vi "Set Theme.vi"(10 "Dark?":bool, 11 "VI in":refnum<vi>) -> ()   [LabVIEW 2019, in "Panther Dashboard.lvlib"]
uses:
  Panther Dashboard.lvlib
  <vilib>/Utility/miscctls.llb/LVTextColorsTypeDef.ctl
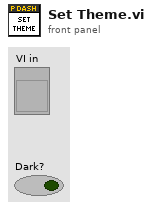
[diagram p1: front panel]
types:
  T1 = typedef "LVTextColorsTypeDef.ctl" = cluster{"Text Color":u32, "Background Color":u32}
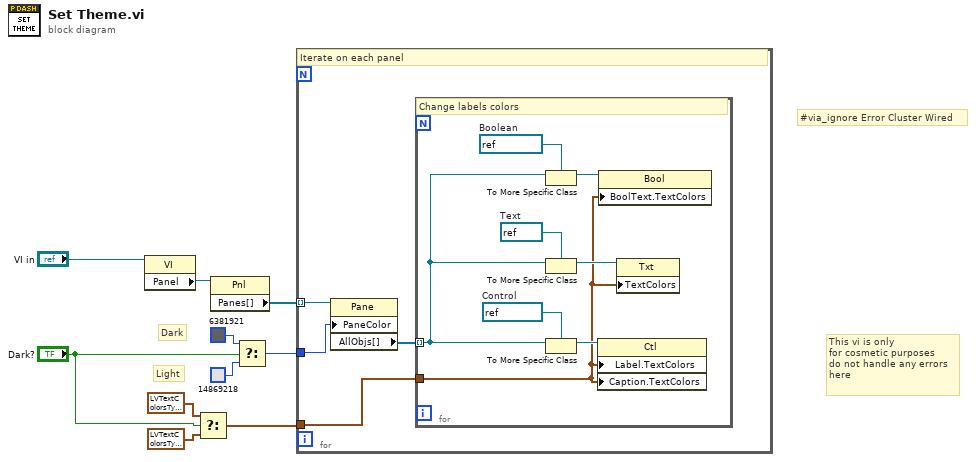
[diagram p0: block diagram]
diagram:
  # "#via_ignore Error Cluster Wired"
  # "This vi is only \nfor cosmetic purposes\ndo not handle any errors\nhere"
  # "Light"
  # "Dark"
  n1 = property class="VI"(reference="VI in") -> ("Panel"=w5:refnum<vi>)  [unwired: 1 in, 2 out]
  n2 = Select(t=T1 {"Text Color"=16448250, "Background Color"=16777216} ("Label.Text Colors"), s="Dark?", f=T1 {"Text Color"=0, "Background Color"=16777216} ("Label.Text Colors")) -> (s? t:f=w2:T1)
  n3 = property class="Pnl"(reference=w5) -> ("Panes[]"=w4:refnum<vi>[])  [unwired: 1 in, 2 out]
  n4 = Select(t=u32 6381921, s="Dark?", f=u32 14869218) -> (s? t:f=w3:u32)
  n5 = for {
    tunnel: w4 -> [w13] mode=indexing
    tunnel: w3 -> [w11]
    tunnel: w2 -> [w14]
    # "Iterate on each panel"
    n6 = property class="Pane"(reference=w13, "PaneColor"=w11) -> ("AllObjs[]"=w12:refnum<vi>[])  [unwired: 1 in, 2 out]
    n7 = for {
      tunnel: w12 -> [w16] mode=indexing
      tunnel: w14 -> [w15]
      w18 = refnum<vi> refnum  # Boolean
      w19 = refnum<vi> refnum  # Text
      w21 = refnum<vi> refnum  # Control
      # "Change labels colors"
      n8 = To More Specific Class(target class=w18, reference=w16) -> (specific class reference=w17:refnum<vi>)  [unwired: 1 in, 1 out]
      n9 = To More Specific Class(target class=w19, reference=w16) -> (specific class reference=w20:refnum<vi>)  [unwired: 1 in, 1 out]
      n10 = To More Specific Class(target class=w21, reference=w16) -> (specific class reference=w22:refnum<vi>)  [unwired: 1 in, 1 out]
      n11 = property class="Ctl"(reference=w22, "Label.TextColors"=w15, "Caption.TextColors"=w15) -> ()  [unwired: 1 in, 2 out]
      n12 = property class="Bool"(reference=w17, "BoolText.TextColors"=w15) -> ()  [unwired: 1 in, 2 out]
      n13 = property class="Txt"(reference=w20, "TextColors"=w15) -> ()  [unwired: 1 in, 2 out]
    }
  }
